vi "XYZ Table Stage Module.vi"(6 "Set/Get":T5=enum."Get", 7 "Action":T1, 8 "Error In":errorcluster, 10 "Axis":enum16{"X Axis", "Y Axis", "Z Axis"}(ring), 11 "Table Stages":T2={"X Stage"={"Position"=0.0, "Is.Enabled?"=FALSE, "Is.Connected?"=FALSE, "Device SN"="45876539", "AccelerationMaximum"=0.0, "VelocityMaximum"=0.0, "Acceleration"=0.0, "Velocity"=0.0, "waitTimeout (ms)"=0, "Model"=enum."None", "Is.Homed?"=FALSE, "MOVE"=FALSE}, "Y Stage"={"Position"=0.0, "Is.Enabled?"=FALSE, "Is.Connected?"=FALSE, "Device SN"="45876539", "AccelerationMaximum"=0.0, "VelocityMaximum"=0.0, "Acceleration"=0.0, "Velocity"=0.0, "waitTimeout (ms)"=0, "Model"=enum."None", "Is.Homed?"=FALSE, "MOVE"=FALSE}, "Z Stage"={"Position"=0.0, "Is.Enabled?"=FALSE, "Is.Connected?"=FALSE, "Device SN"="45876539", "AccelerationMaximum"=0.0, "VelocityMaximum"=0.0, "Acceleration"=0.0, "Velocity"=0.0, "waitTimeout (ms)"=0, "Model"=enum."None", "Is.Homed?"=FALSE, "MOVE"=FALSE}, "Attenuator"={"Position"=0.0, "Is.Enabled?"=FALSE, "Is.Connected?"=FALSE, "Device SN"="45876539", "AccelerationMaximum"=0.0, "VelocityMaximum"=0.0, "Acceleration"=0.0, "Velocity"=0.0, "waitTimeout (ms)"=0, "Model"=enum."None", "Is.Homed?"=FALSE, "MOVE"=FALSE}}) -> (0 "Error Out":errorcluster, 3 "Table Stages [out]":T2={"X Stage"={"Position"=0.0, "Is.Enabled?"=FALSE, "Is.Connected?"=FALSE, "Device SN"="45876539", "AccelerationMaximum"=0.0, "VelocityMaximum"=0.0, "Acceleration"=0.0, "Velocity"=0.0, "waitTimeout (ms)"=0, "Model"=enum."None", "Is.Homed?"=FALSE, "MOVE"=FALSE}, "Y Stage"={"Position"=0.0, "Is.Enabled?"=FALSE, "Is.Connected?"=FALSE, "Device SN"="45876539", "AccelerationMaximum"=0.0, "VelocityMaximum"=0.0, "Acceleration"=0.0, "Velocity"=0.0, "waitTimeout (ms)"=0, "Model"=enum."None", "Is.Homed?"=FALSE, "MOVE"=FALSE}, "Z Stage"={"Position"=0.0, "Is.Enabled?"=FALSE, "Is.Connected?"=FALSE, "Device SN"="45876539", "AccelerationMaximum"=0.0, "VelocityMaximum"=0.0, "Acceleration"=0.0, "Velocity"=0.0, "waitTimeout (ms)"=0, "Model"=enum."None", "Is.Homed?"=FALSE, "MOVE"=FALSE}, "Attenuator"={"Position"=0.0, "Is.Enabled?"=FALSE, "Is.Connected?"=FALSE, "Device SN"="45876539", "AccelerationMaximum"=0.0, "VelocityMaximum"=0.0, "Acceleration"=0.0, "Velocity"=0.0, "waitTimeout (ms)"=0, "Model"=enum."None", "Is.Homed?"=FALSE, "MOVE"=FALSE}})   [LabVIEW 2018]
uses:
  General/Controls/Set Get Controls.ctl
  General/Controls/Translation Stage Parameters.ctl
  Controls/Translation Stage Cluster.ctl
  General/Controls/Translation Stage Types.ctl
  Controls/Motion Translation Module Control2.ctl
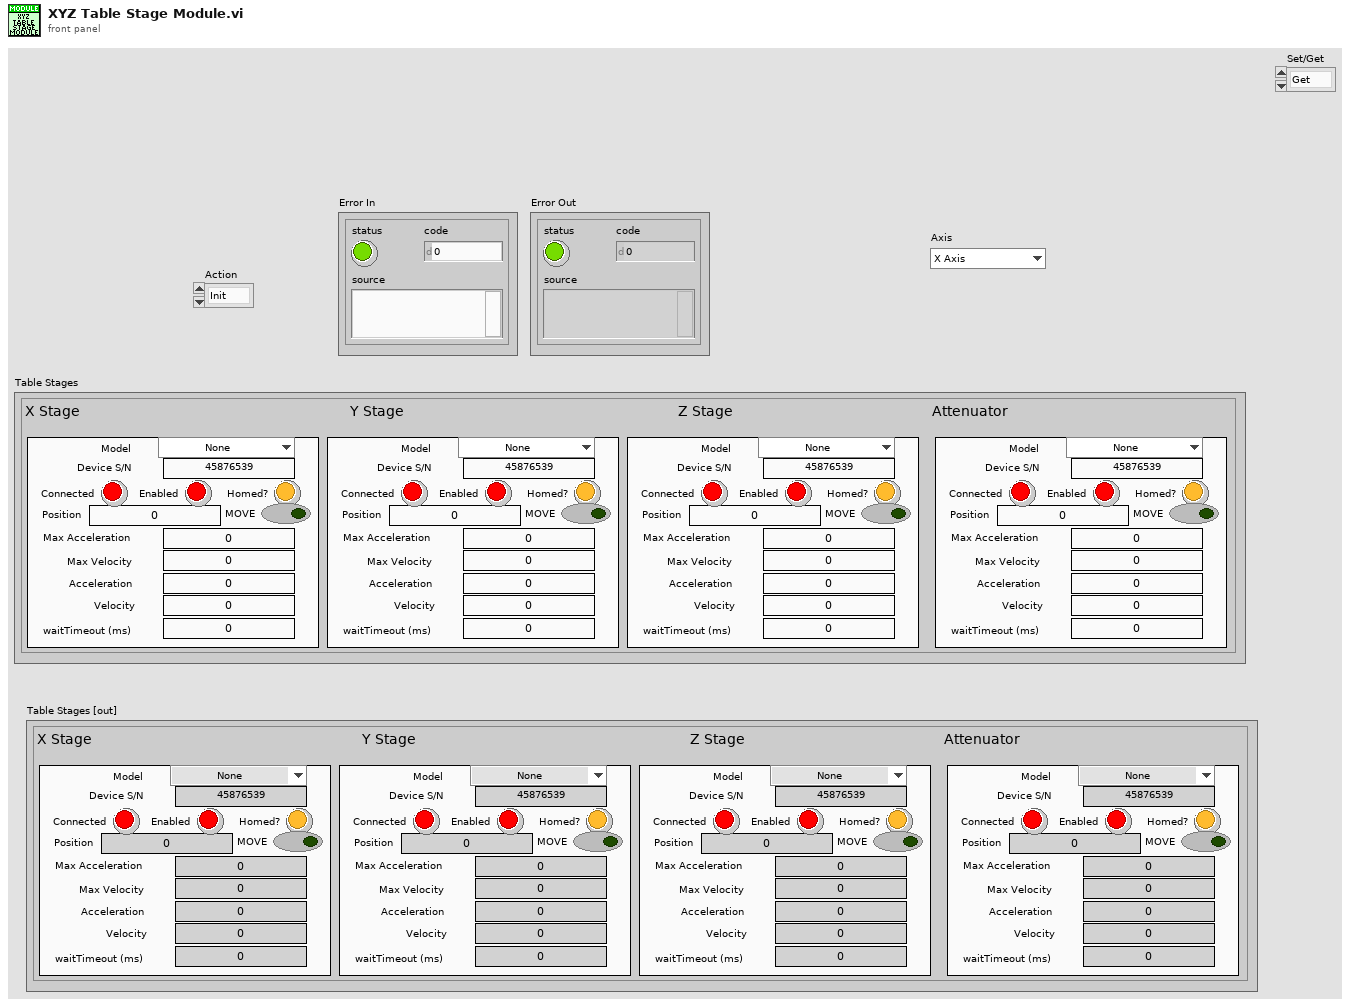
[diagram p1: front panel]
types:
  T1 = typedef "Motion Translation Module Control2.ctl" = enum16{"Init", "Home", "Status", "Velocity/Accel", "Position", "Jog", "Stop", "Uninit", "Enable", "Disable"}
  T2 = typedef "Translation Stage Parameters.ctl" = cluster{"X Stage":T3, "Y Stage":T3, "Z Stage":T3, "Attenuator":T3}
  T3 = typedef "Translation Stage Cluster.ctl" = cluster{"Position":dbl, "Is.Enabled?":bool, "Is.Connected?":bool, "Device SN":string, "AccelerationMaximum":dbl, "VelocityMaximum":dbl, "Acceleration":dbl, "Velocity":dbl, "waitTimeout (ms)":i32, "Model":T4, "Is.Homed?":bool, "MOVE":bool}
  T4 = typedef "Translation Stage Types.ctl" = enum16{"None", "Thorlabs LTS", "Thorlabs MLJ"}
  T5 = typedef "Set Get Controls.ctl" = enum16{"Set", "Get"}
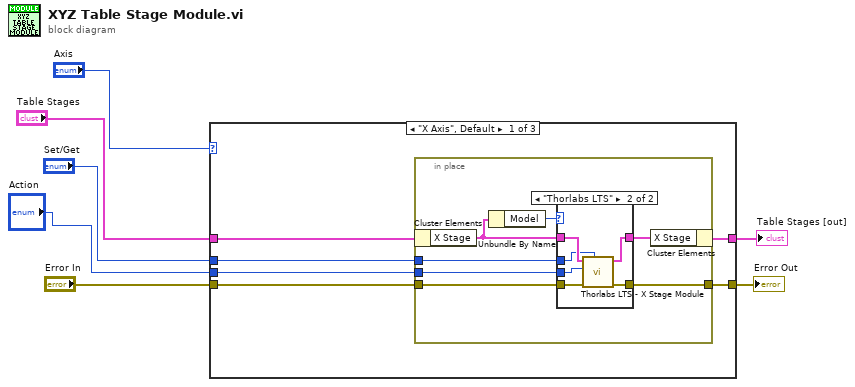
[diagram p0: block diagram]
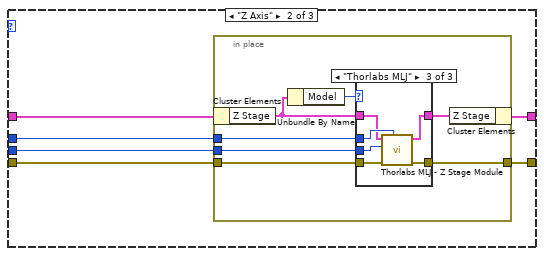
[diagram p3: hidden frame]
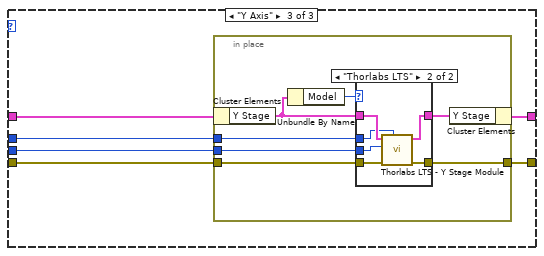
[diagram p6: hidden frame]
diagram:
  n1 = case shown="\"X Axis\", Default" "Axis" {
    tunnel: "Set/Get" -> [w10 w32 w54]
    tunnel: "Error In" -> [w13 w34 w57]
    tunnel: "Action" -> [w11 w31 w55]
    tunnel: [w12 w33 w56] -> w6
    tunnel: "Table Stages" -> [w9 w30 w53]
    tunnel: [w8 w29 w52] -> w2
    frame "X Axis", Default {
      n2 = in-place {
        in-place-border: w13 -> [w20]
        in-place-border: [w19] -> w12
        in-place-border: w11 -> [w18]
        in-place-border: w10 -> [w17]
        n3 = in-place-cluster #1(w9) -> ("X Stage"=w15:T3)
        n4 = Unbundle By Name(w15) -> ("Model"=w16:T4)
        n5 = case shown="\"Thorlabs LTS\"" w16 {
          tunnel: w20 -> [w22 w28]
          tunnel: [w22 w27] -> w19
          tunnel: w15 -> [w21 w26]
          tunnel: w18 -> [_ w25]
          tunnel: [w21 w24] -> w14
          tunnel: w17 -> [_ w23]
          frame "None", Default {
          }
          frame "Thorlabs LTS" {
            n6 = call "Thorlabs LTS - X Stage Module.vi"("Set/Get"=w23, "Error In"=w28, "Action"=w25, "Cluster In"=w26) -> ("Error Out"=w27:errorcluster, "Cluster Out"=w24:T3)  [unwired: 6 in]
          }
        }
        n7 = in-place-cluster #1("X Stage"=w14) -> (w8:T2)
      }
    }
    frame "Z Axis" {
      n8 = in-place {
        in-place-border: w34 -> [w41]
        in-place-border: [w40] -> w33
        in-place-border: w32 -> [w39]
        in-place-border: w31 -> [w38]
        n9 = in-place-cluster #2(w30) -> ("Z Stage"=w36:T3)
        n10 = Unbundle By Name(w36) -> ("Model"=w37:T4)
        n11 = case shown="\"Thorlabs MLJ\"" w37 {
          tunnel: w41 -> [w43 w45 w51]
          tunnel: [w43 w45 w50] -> w40
          tunnel: [w42 w44 w49] -> w35
          tunnel: w39 -> [_ _ w48]
          tunnel: w38 -> [_ _ w47]
          tunnel: w36 -> [w42 w44 w46]
          frame "None", Default {
          }
          frame "Thorlabs LTS" {
          }
          frame "Thorlabs MLJ" {
            n12 = call "Thorlabs MLJ - Z Stage Module.vi"("Set/Get"=w48, "Error In"=w51, "Action"=w47, "Cluster In"=w46) -> ("Error Out"=w50:errorcluster, "Cluster Out"=w49:T3)  [unwired: 6 in]
          }
        }
        n13 = in-place-cluster #2("Z Stage"=w35) -> (w29:T2)
      }
    }
    frame "Y Axis" {
      n14 = in-place {
        in-place-border: w57 -> [w64]
        in-place-border: [w63] -> w56
        in-place-border: w55 -> [w62]
        in-place-border: w54 -> [w61]
        n15 = in-place-cluster #3(w53) -> ("Y Stage"=w59:T3)
        n16 = Unbundle By Name(w59) -> ("Model"=w60:T4)
        n17 = case shown="\"Thorlabs LTS\"" w60 {
          tunnel: w64 -> [w66 w72]
          tunnel: [w66 w71] -> w63
          tunnel: [w65 w70] -> w58
          tunnel: w59 -> [w65 w69]
          tunnel: w62 -> [_ w68]
          tunnel: w61 -> [_ w67]
          frame "None", Default {
          }
          frame "Thorlabs LTS" {
            n18 = call "Thorlabs LTS - Y Stage Module.vi"("Set/Get"=w67, "Error In"=w72, "Action"=w68, "Cluster In"=w69) -> ("Error Out"=w71:errorcluster, "Cluster Out"=w70:T3)  [unwired: 6 in]
          }
        }
        n19 = in-place-cluster #3("Y Stage"=w58) -> (w52:T2)
      }
    }
  }
  "Error Out" <- w6
  "Table Stages [out]" <- w2
